vi "iterate.vi"(8 "error in (no error)":errorcluster, 11 "DL090211ImageAssemblerScaffold in":refnum<class "ImageAssemblerDL090211Scaffold.lvclass">) -> (0 "error out":errorcluster, 2 "finished?":bool, 3 "DL090211ImageAssemblerScaffold out":refnum<class "ImageAssemblerDL090211Scaffold.lvclass">)   [LabVIEW 2010, in "ImageAssemblerDL090211Scaffold.lvclass"]
uses:
  ImageAssemblerDL090211Scaffold.lvclass
  ImageAssemblerDL090211Scaffold.lvclass/ImageAssemblerDL090211Scaffold.ctl
  common/classes/GenericComponent/GenericComponent/class_data.vi
  common/classes/GenericComponent/GenericComponent/GenericComponent.lvclass
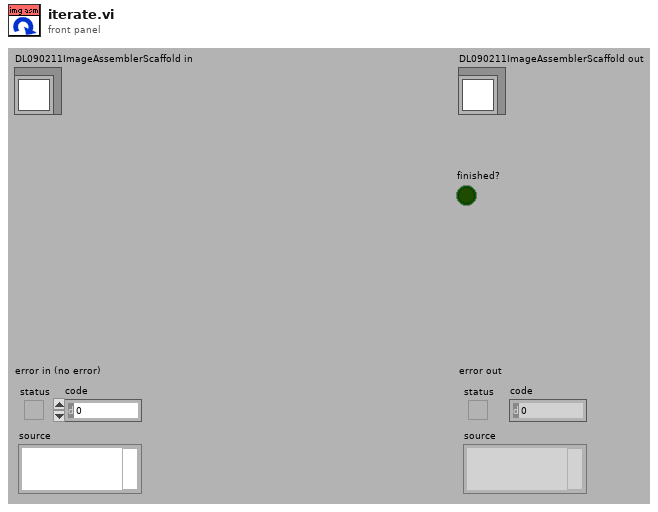
[diagram p1: front panel]
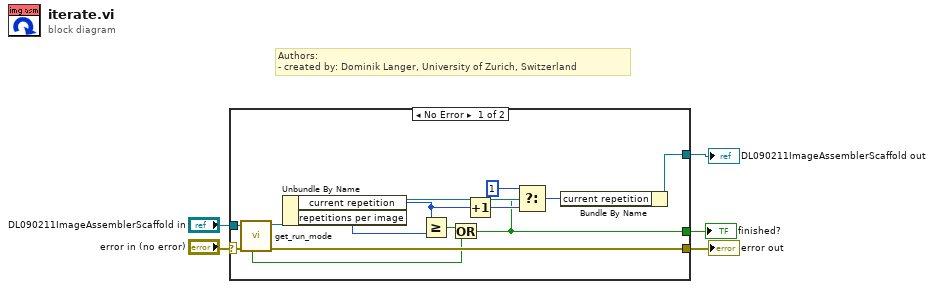
[diagram p0: block diagram]
diagram:
  # "Authors: \n- created by: Dominik Langer, University of Zurich, Switzerland"
  n1 = case shown="No Error" "error in (no error)" {
    selector: "error in (no error)" -> [w12 w20]
    tunnel: [w11 w20] -> w4
    tunnel: [w18 w19] -> w2
    tunnel: "DL090211ImageAssemblerScaffold in" -> [w10 w19]
    tunnel: [w6 _] -> w1
    frame No Error {
      n2 = call "get_run_mode.vi"("error in (no error)"=w12, "GenericPlugin in"=w10) -> ("error out"=w11:errorcluster, "GenericPlugin out"=w9:refnum<class "ImageAssemblerDL090211Scaffold.lvclass">, "is free run?"=w8:bool)  [unwired: 5 in, 2 out]
      n3 = Unbundle By Name(w9) -> ("current repetition"=w14:i32, "repetitions per image"=w17:i32)
      n4 = Greater Or Equal?(x=w14, y=w17) -> (x >= y?=w7:bool)
      n5 = Or(x=w7, y=w8) -> (x .or. y?=w6:bool)
      n6 = Increment(x=w14) -> (x+1=w15:i32)
      n7 = Select(t=1, s=w6, f=w15) -> (s? t:f=w13:i32)
      n8 = Bundle By Name(cluster=w9, "current repetition"=w13) -> (w18:refnum<class "ImageAssemblerDL090211Scaffold.lvclass">)
    }
    frame Error {
    }
  }
  "error out" <- w4
  "DL090211ImageAssemblerScaffold out" <- w2
  "finished?" <- w1
